vi "Write URI.vi"(8 "error in (no error)":errorcluster, 10 "URI":string, 11 "WebSocket Server in":refnum<class "WebSocket Server.lvclass">) -> (0 "error out":errorcluster, 3 "WebSocket Server out":refnum<class "WebSocket Server.lvclass">)   [LabVIEW 2016, in "WebSocket Actor.lvlib" / "WebSocket Server.lvclass"]
uses:
  WebSocket Server.lvclass
  WebSocket Server.lvclass/WebSocket Server.ctl
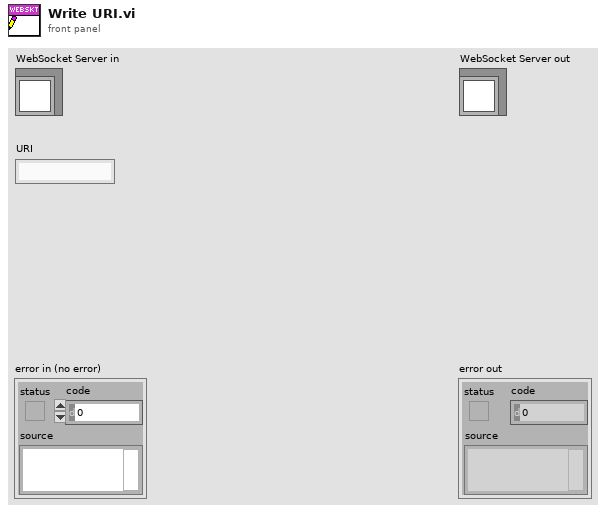
[diagram p1: front panel]
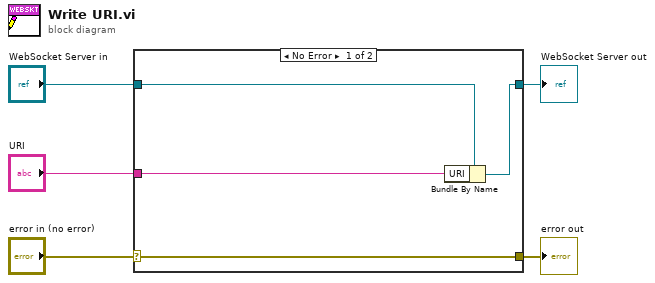
[diagram p0: block diagram]
diagram:
  n1 = case shown="No Error" "error in (no error)" {
    selector: "error in (no error)" -> [w9 w10]
    tunnel: [w9 w10] -> w4
    tunnel: [w7 w11] -> w2
    tunnel: "WebSocket Server in" -> [w8 w11]
    tunnel: "URI" -> [w6 _]
    frame No Error {
      n2 = Bundle By Name(cluster=w8, "URI"=w6) -> (w7:refnum<class "WebSocket Server.lvclass">)
    }
    frame Error {
    }
  }
  "error out" <- w4
  "WebSocket Server out" <- w2
